vi "Is Transmit Ready.vi"(6 "Buffer size":i32=16384 format="0x%x (0d%d)", 8 "error in (no error)":errorcluster, 10 "Samples to transmit":i32=1024, 11 "RP Instrument in":refnum<class "RP Instrument.lvclass">) -> (0 "error out":errorcluster, 1 "Unused buffer":i32, 2 "Transmit Ready":bool, 3 "RP Instrument out":refnum<class "RP Instrument.lvclass">)   [LabVIEW 2016, in "RP Instrument.lvclass"]
uses:
  RP Instrument.lvclass
  RP Status Offsets.ctl
  RP Instrument.lvclass/RP Instrument.ctl
  RP Communicator/RP Communicator.lvclass
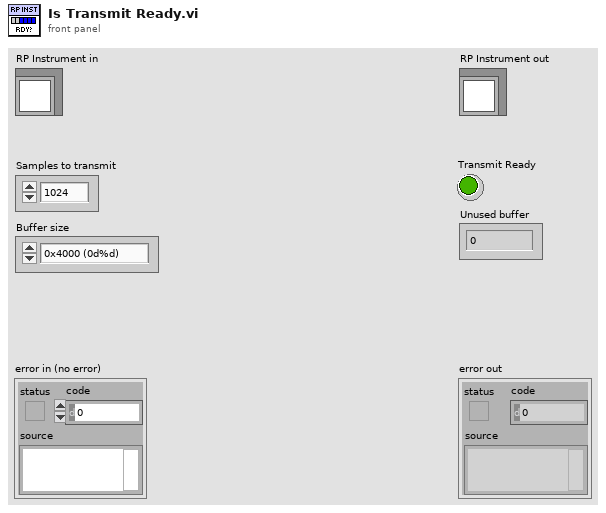
[diagram p1: front panel]
types:
  T1 = typedef "RP Status Offsets.ctl" = u16
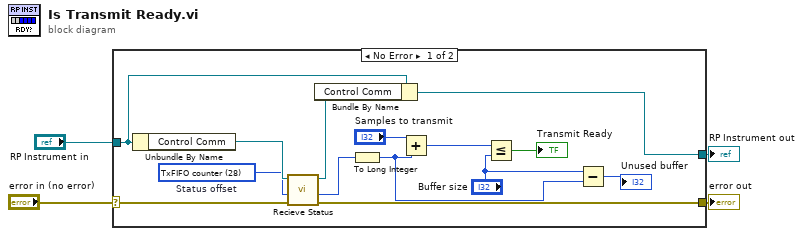
[diagram p0: block diagram]
diagram:
  n1 = case shown="No Error" "error in (no error)" {
    selector: "error in (no error)" -> [w11 w20]
    tunnel: [w10 w20] -> w3
    tunnel: [w13 w19] -> w1
    tunnel: "RP Instrument in" -> [w18 w19]
    frame No Error {
      w16 = T1 28 items=["Writer address"=0, "Record start position"=4, "Trig state etc."=8, "RxFIFO counter"=24, "TxFIFO counter"=28]  # Status offset
      n2 = Unbundle By Name(w18) -> ("Control Comm"=w17:refnum<class "RP Communicator.lvclass">)
      n3 = call-dynamic "Recieve Status.vi"("error in (no error)"=w11, "Status offset"=w16, "RP Communicator in"=w17) -> ("error out"=w10:errorcluster, "Status response"=w15:u32, "RP Communicator out"=w12:refnum<class "RP Communicator.lvclass">)  [unwired: 6 in]
      n4 = Bundle By Name(cluster=w18, "Control Comm"=w12) -> (w13:refnum<class "RP Instrument.lvclass">)
      n5 = To Long Integer(number=w15) -> (32bit integer=w6:i32)
      n6 = Add(x="Samples to transmit", y=w6) -> (x+y=w7:i32)
      n7 = Less Or Equal?(x=w7, y="Buffer size") -> (x <= y?=→"Transmit Ready":bool)
      n8 = Subtract(x="Buffer size", y=w6) -> (x-y=→"Unused buffer":i32)
    }
    frame Error {
    }
  }
  "error out" <- w3
  "RP Instrument out" <- w1
